vi "Merge Error.vi"(10 "Error":errorcluster, 11 "Hello World Event in":refnum<class "Hello World Event.lvclass">) -> (3 "Hello World Event out":refnum<class "Hello World Event.lvclass">)   [LabVIEW 2021, in "Hello World Event.lvlib" / "Hello World Event.lvclass"]
uses:
  Hello World Event.lvclass
  Hello World Event.lvclass/Hello World Event.ctl
  jettl/Event jettl/Event jettl.lvclass
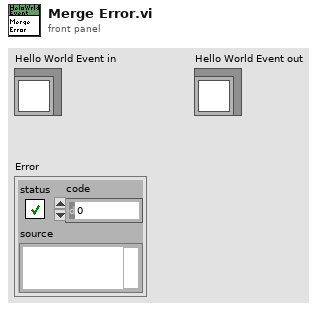
[diagram p1: front panel]
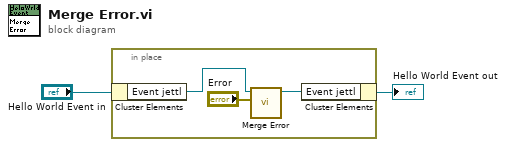
[diagram p0: block diagram]
diagram:
  n1 = in-place {
    n2 = in-place-cluster #1("Hello World Event in") -> ("Event jettl"=w5:refnum<class "Event jettl.lvclass">)
    n3 = call-dynamic "Merge Error.vi"("Error"="Error", "Merge Error in"=w5) -> ("Merge Error out"=w4:refnum<class "Event jettl.lvclass">)  [unwired: 9 in]
    n4 = in-place-cluster #1("Event jettl"=w4) -> (→"Hello World Event out":refnum<class "Hello World Event.lvclass">)
  }
